vi "PING网络状态.vi"() -> ()   [LabVIEW 2016, in "环境动力监测库.lvlib"]
panel:
  out "网络状态":bool
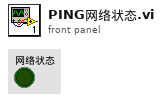
[diagram p1: front panel]
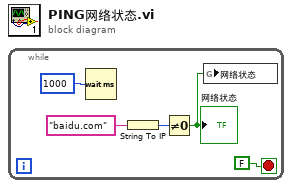
[diagram p0: block diagram]
diagram:
  n1 = while {
    stop <- FALSE stop-if-true
    n2 = Wait (ms)(milliseconds to wait=u32 1000 ("等待时间（毫秒）")) -> ()  [unwired: 1 out]
    n3 = String To IP(1:"baidu.com" ("地址")) -> (0:w4:u32)
    n4 = Not Equal To 0?(x=w4) -> (x != 0?=w1:bool)
    "网络状态" <- w1
    n5 = global write "内部交互全局变量.vi" "网络状态"(w1) -> ()
  }
